vi "Updater Setup DIAdem 2012.vi"(8 "error in (no error)":errorcluster) -> (0 "error out":errorcluster)   [LabVIEW 2011]
uses:
  <vilib>/registry/registry.llb/Read Registry Value Simple STR.vi
  Summitek EXT/OpenG EXT/file/file.llb/File Exists - Scalar__ogtk.vi
  Summitek EXT/OpenG EXT/largefile/largefile.llb/LF Write File (STR)__ogtk.vi
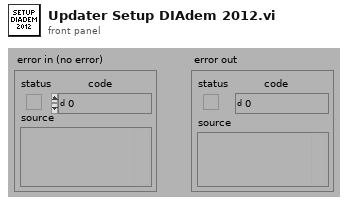
[diagram p1: front panel]
types:
  T1 = enum16{"open", "replace", "create", "open or create", "replace or create", "replace or create with confirmation"}
  T2 = typedef "Registry refnum.ctl" = refnum<k1>
  T3 = typedef "DIAdem Reference.ctl" = cluster{"ToCommand Reference":refnum<k7>, "ToDataSheet Reference":refnum<k7>}
  T4 = cluster{"ToCommand Reference":bool, "ToDataSheet Reference":bool}
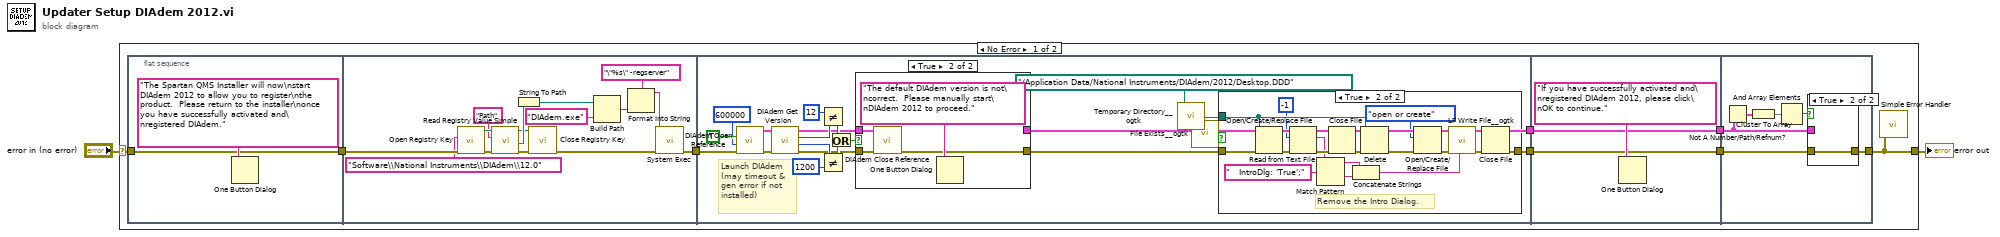
[diagram p0: block diagram]
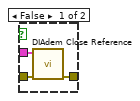
[diagram p4: hidden frame]
diagram:
  n1 = case shown="No Error" "error in (no error)" {
    selector: "error in (no error)" -> [w3 w89]
    tunnel: [w4 w89] -> w2
    frame No Error {
      n2 = flat-sequence {
        tunnel: [w11] -> w10
        tunnel: w3 -> [w11]
        tunnel: w10 -> [w27]
        tunnel: [w17] -> w9
        tunnel: w9 -> [w31]
        tunnel: [w30] -> w8
        tunnel: [w34] -> w7
        tunnel: w8 -> [w77]
        tunnel: [w77] -> w6
        tunnel: w7 -> [w76]
        tunnel: [w76] -> w5
        tunnel: [w83] -> w4
        tunnel: w6 -> [w84]
        tunnel: w5 -> [w82]
        frame #0 {
          n3 = One Button Dialog(message="The Spartan QMS Installer will now\nstart DIAdem 2012 to allow you to register\nthe product.  Please return to the installer\nonce you have successfully activated and\nregistered DIAdem.") -> ()  [unwired: 1 in, 1 out]
        }
        frame #1 {
          n4 = call <vilib>:"Open Registry Key.vi"("error in (no error)"=w27, "subkey"="Software\\National Instruments\\DIAdem\\12.0") -> ("error out"=w26:errorcluster, "refnum out"=w25:T2)  [unwired: 8 in]
          n5 = call-poly <vilib>:"Read Registry Value Simple.vi"("error in (no error)"=w26, "value"="Path" ("subkey"), "refnum"=w25) -> ("error out"=w21:errorcluster, "String/Binary data"=w23:string, "refnum out"=w22:T2)  [unwired: 3 in, 1 out]
          n6 = String To Path(string=w23) -> (path=w20:path)
          n7 = call <vilib>:"Close Registry Key.vi"("error in (no error)"=w21, "refnum"=w22) -> ("error out"=w18:errorcluster)  [unwired: 5 in]
          n8 = Build Path(base path=w20, name or relative path="DIAdem.exe" ("subkey")) -> (appended path=w15:path)
          n9 = Format Into String(format string="\"%s\" -regserver", w15) -> (resulting string=w14:string)  [unwired: 2 in, 1 out]
          n10 = call <vilib>:"System Exec.vi"("error in (no error)"=w18, "command line"=w14) -> ("error out"=w17:errorcluster)  [unwired: 6 in, 3 out]
        }
        frame #2 {
          # "Launch DIAdem\n(may timeout &\ngen error if not\ninstalled)"
          n11 = call "DIAdem Open Reference.vi"("error in (no error)"=w31, "Timeout (ms)"=u32 600000, "Show Environment (F)"=TRUE) -> ("error out"=w46:errorcluster, "DIAdem Reference"=w45:T3)  [unwired: 1 in, 6 out]
          n12 = call "DIAdem Get Version.vi"("error in (no error)"=w46, "DIAdem Reference"=w45) -> ("error out"=w35:errorcluster, "Revision"=w41:i32, "Version"=w43:i32, "DIAdem Reference"=w36:T3)  [unwired: 5 in]
          n13 = Not Equal?(x=12, y=w43) -> (x != y?=w39:bool)
          n14 = Not Equal?(x=w41, y=1200) -> (x != y?=w38:bool)
          n15 = Or(x=w39, y=w38) -> (x .or. y?=w37:bool)
          n16 = case shown="True" w37 {
            tunnel: w36 -> [w71 w75]
            tunnel: w35 -> [w70 w74]
            tunnel: [w70 w72] -> w29
            tunnel: [w71 _] -> w34
            frame False {
            }
            frame True {
              n17 = call <vilib>:"DIAdem Close Reference.vi"("error in (no error)"=w74, "DIAdem Reference"=w75) -> ("error out"=w72:errorcluster)  [unwired: 9 in]
              n18 = One Button Dialog(message="The default DIAdem version is not\ncorrect.  Please manually start\nDIAdem 2012 to proceed.") -> ()  [unwired: 1 in, 1 out]
            }
          }
          n19 = call "Temporary Directory__ogtk.vi"("Relative path (.)"=path "../Application Data/National Instruments/DIAdem/2012/Desktop.DDD") -> ("Temporary Directory (+ Relative)"=w33:path)
          n20 = call-poly "File Exists__ogtk.vi"("file path"=w33) -> ("exists"=w32:bool)  [unwired: 6 in, 1 out]
          n21 = case shown="True" w32 {
            tunnel: w29 -> [w48 w67]
            tunnel: [w48 w59] -> w30
            tunnel: w33 -> [_ w52]
            frame False {
              # "File does not exist."
            }
            frame True {
              # "Remove the Intro Dialog."
              n22 = Open/Create/Replace File(file path (use dialog)=w52, error in=w67) -> (refnum out=w56:refnum<file>, error out=w66:errorcluster)  [unwired: 4 in, 1 out]
              n23 = Read from Text File(file (use dialog)=w56, count=-1, error in=w66) -> (refnum out=w64:refnum<file>, text=w50:string, error out=w65:errorcluster)  [unwired: 1 in, 1 out]
              n24 = Match Pattern(string=w50, regular expression="   IntroDlg: 'True';") -> (before substring=w69:string, after substring=w68:string)  [unwired: 1 in, 2 out]
              n25 = Close File(refnum=w64, error in=w65) -> (error out=w54:errorcluster)  [unwired: 1 out]
              n26 = Concatenate Strings(w69, w68) -> (w58:string)
              n27 = Delete(path (use dialog)=w52, error in=w54) -> (deleted path=w51:path, error out=w53:errorcluster)  [unwired: 3 in, 1 out]
              n28 = Open/Create/Replace File(file path (use dialog)=w51, error in=w53, operation (0:open)=T1."open or create") -> (refnum out=w61:refnum<file>, error out=w62:errorcluster)  [unwired: 3 in, 1 out]
              n29 = call-poly "LF Write File__ogtk.vi"("data"=w58, "error in (no error)"=w62, "refnum"=w61) -> ("error out"=w63:errorcluster, "refnum out"=w60:refnum<file>)  [unwired: 5 in, 1 out]
              n30 = Close File(refnum=w60, error in=w63) -> (error out=w59:errorcluster)  [unwired: 1 out]
            }
          }
        }
        frame #3 {
          n31 = One Button Dialog(message="If you have successfully activated and\nregistered DIAdem 2012, please click\nOK to continue.") -> ()  [unwired: 1 in, 1 out]
        }
        frame #4 {
          n32 = Not A Number/Path/Refnum?(number/path/refnum=w82) -> (NaN/Path/Refnum?=w81:T4)
          n33 = Cluster To Array(cluster=w81) -> (array=w80:bool[])
          n34 = And Array Elements(Boolean array=w80) -> (logical AND=w79:bool)
          n35 = case shown="True" w79 {
            tunnel: w84 -> [w87 w88]
            tunnel: [w86 w88] -> w83
            tunnel: w82 -> [w85 _]
            frame False {
              n36 = call <vilib>:"DIAdem Close Reference.vi"("error in (no error)"=w87, "DIAdem Reference"=w85) -> ("error out"=w86:errorcluster)  [unwired: 9 in]
            }
            frame True {
            }
          }
        }
      }
      n37 = call <vilib>:"Simple Error Handler.vi"("error in (no error)"=w4) -> ()  [unwired: 4 in, 5 out]
    }
    frame Error {
    }
  }
  "error out" <- w2
